vi "Memory.Pointer.Advanced Copy.Safe.vi"(0 "src pointer in":refnum<class "Memory.Pointer.lvclass">, 1 "dst width":u64 format="%d bytes", 2 "src width":u64 format="%d bytes", 3 "byte order (big-endian)":enum16{"big-endian", "little-endian"}(ring), 5 "dst pointer in":refnum<class "Memory.Pointer.lvclass">, 7 "src offset (0)":u64 format="%d bytes", 9 "dst offset (0)":u64 format="%d bytes", 11 "error in (no error)":errorcluster, 12 "clear dst bytes? (T)":bool=TRUE) -> (4 "src pointer out":refnum<class "Memory.Pointer.lvclass">, 6 "dst pointer out":refnum<class "Memory.Pointer.lvclass">, 15 "error out":errorcluster)   [LabVIEW 2016, in "Memory.lvlib" / "Memory.Pointer.lvclass"]
doc: "Moves bytes of data from the <b>src pointer</b> at <b>src offset</b> to the <b>dst pointer</b> at <b>dst offset</b> using the <b>byte order</b> specified. <b>src width</b> and <b>dst width</b> are used to determine how many bytes to move, as well as where the bytes should be read from/written to in memory. For example, to type cast a DBL to a U16, src width would be 8 bytes and dst width would be 2 bytes.\n\nThe optional argument <b>clear dst bytes</b> will clear the subset of bytes within <b>dst pointer</b> before moving data from the <b>src pointer</b>. This is required when type casting from a smaller type to a larger type, as the larger type may have non-zero bytes that will not get overwritten. This argument can be set the FALSE when casting larger types down to smaller types.\n\n<b>Note:</b> This VI is <b>safe</b>, meaning it performs null pointer and bounds checks to prevent invalid memory access."
uses:
  Memory.Pointer.lvclass
  Memory.Pointer.lvclass/Memory.Pointer.ctl
  Memory.Pointer.Errors.vi
  Memory.Pointer.Errors.Null Pointer.vi
  Memory.Pointer.Get Address.vi
  Memory.Pointer.Errors.Out of Bounds.vi
  Memory.Pointer.Get Size.vi
  Memory.Pointer.Advanced Copy.Adjust Parameters.vi
  Memory.Pointer.Clear Subset.Unsafe.vi
  Memory.Pointer.Errors.Create Error.vi
  Submodules/SEH/Source/VIs/Static Error Handling.Source Buffer.Write.String.vi
  Memory.Pointer.Errors.Write Pointer Size.vi
  Submodules/SEH/Source/VIs/Static Error Handling.Source Buffer.Write.Numeric.Scalar.Base10.vi
  Submodules/SEH/Source/VIs/Static Error Handling.Source Buffer.Write.Numeric.Scalar.Base10 (U64).vi
  Submodules/SEH/Source/VIs/Static Error Handling.Error Cluster Constant.vi
  Submodules/SEH/Source/VIs/Static Error Handling.Error Cluster Constant (256B).vi
  Submodules/SEH/Source/VIs/Static Error Handling.Parameters.Status.Set.vi
  Submodules/SEH/Source/VIs/Static Error Handling.Parameters.Code.Set.vi
  Submodules/SEH/Source/VIs/Static Error Handling.Parameters.VI Source.Set.vi
  Constants/Memory.Constants.vi
  Constants/Memory.Constants.Library Name.vi
  Memory.Pointer.Errors.Get Info.vi
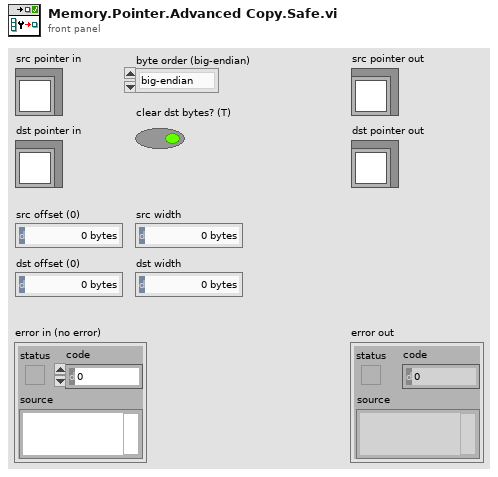
[diagram p1: front panel]
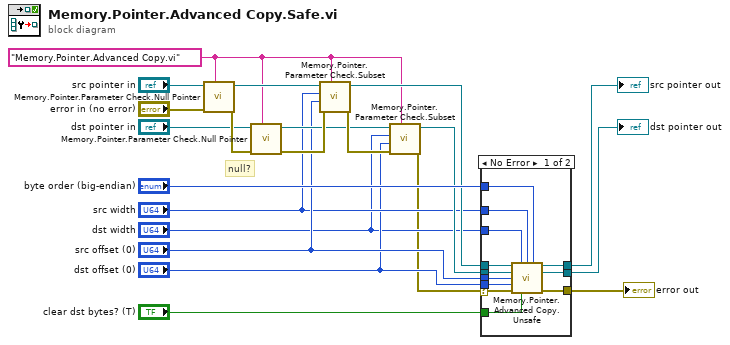
[diagram p0: block diagram]
diagram:
  w6 = "Memory.Pointer.Advanced Copy.vi" ("source vi name")
  # "null?"
  n1 = call "Memory.Pointer.Parameter Check.Null Pointer.vi"("source vi name"=w6, "error in (no error)"="error in (no error)", "Pointer in"="src pointer in") -> ("error out"=w20:errorcluster, "Pointer out"=w12:refnum<class "Memory.Pointer.lvclass">)  [unwired: 7 in]
  n2 = call "Memory.Pointer.Parameter Check.Null Pointer.vi"("source vi name"=w6, "error in (no error)"=w20, "Pointer in"="dst pointer in") -> ("error out"=w19:errorcluster, "Pointer out"=w11:refnum<class "Memory.Pointer.lvclass">)  [unwired: 7 in]
  n3 = call "Memory.Pointer.Parameter Check.Subset.vi"("source vi name"=w6, "error in (no error)"=w19, "offset (0)"="src offset (0)", "length"="src width", "Pointer in"=w12) -> ("error out"=w21:errorcluster, "Pointer out"=w9:refnum<class "Memory.Pointer.lvclass">)  [unwired: 3 in, 2 out]
  n4 = call "Memory.Pointer.Parameter Check.Subset.vi"("source vi name"=w6, "error in (no error)"=w21, "offset (0)"="dst offset (0)", "length"="dst width", "Pointer in"=w11) -> ("error out"=w1:errorcluster, "Pointer out"=w10:refnum<class "Memory.Pointer.lvclass">)  [unwired: 3 in, 2 out]
  n5 = case shown="No Error" w1 {
    selector: w1 -> [w22 w34]
    tunnel: [w33 w34] -> w17
    tunnel: "byte order (big-endian)" -> [w32 _]
    tunnel: "clear dst bytes? (T)" -> [w31 _]
    tunnel: w10 -> [w30 w35]
    tunnel: w9 -> [w29 w36]
    tunnel: [w28 w35] -> w8
    tunnel: [w27 w36] -> w7
    tunnel: "src offset (0)" -> [w26 _]
    tunnel: "src width" -> [w25 _]
    tunnel: "dst offset (0)" -> [w24 _]
    tunnel: "dst width" -> [w23 _]
    frame No Error {
      n6 = call "Memory.Pointer.Advanced Copy.Unsafe.vi"("src pointer in"=w29, "dst width"=w23, "src width"=w25, "byte order (big-endian)"=w32, "dst pointer in"=w30, "src offset (0)"=w26, "dst offset (0)"=w24, "error in (no error)"=w22, "clear dst bytes? (T)"=w31) -> ("src pointer out"=w27:refnum<class "Memory.Pointer.lvclass">, "dst pointer out"=w28:refnum<class "Memory.Pointer.lvclass">, "error out"=w33:errorcluster)  [unwired: 4 in]
    }
    frame Error {
    }
  }
  "error out" <- w17
  "src pointer out" <- w7
  "dst pointer out" <- w8
